vi "MOV_C-887.vi"(0 "System no.":i32=1 min=1 max=4 step=1, 2 "Axes to move":string[](array[string]), 3 "Position values":dbl[](array[numeric]) format="%.6f", 4 "No.of digits":i16=4, 5 "error in":errorcluster) -> (19 "error out":errorcluster)   [LabVIEW 2020]
doc: "GCS 3.0\n=====\n\nMOV (Start Absolute Motion)\n\nDescription\nSets absolute target positions for the specified axes and starts the motion to these target \npositions.\nAll axes specified in the command start the motion simultaneously.\nDuring motion, a new motion command sets the target to a new value and the old value may \nnever be reached.\n\nFormat\nMOV{ <AxisID> <Position>}\n\nArguments\n<AxisID>\nAn axis of the controller\nThe response to USG? CMD MOV indicates in the #Related Units block for which axes the \ncommand can be used.\nPossible values: Alias of the axis (p. 94) \n<Position>\nAbsolute target position in physical units\nThe data format is float.\nPossible values: Dependent on the permitted travel range of the axis\n\nResponse\nnone\n\nExample\n>>MOV?\n<<AXIS_1=0.0\n<<AXIS_2=0.0\n>>MOV AXIS_1 20 AXIS_2 40\n>>MOV?\n<<AXIS_1=20.000000000000000\n<<AXIS_2=40.000000000000000\n>>POS?\n<<AXIS_1=19.999494552\n<<AXIS_2=40.000494553\n\nNotes\nMotion is only executed if the following conditions are fulfilled for all specified axes:\n- The axis is in the Operation enabled state.\n- The mode of operation is set to Closed-Loop Position (0x2).\n- The target position is within the currently valid limits.\nFor further details, see \"Drive State Machine\" (p. 101) and the status register of the axis (p. 97). \nThe STV? command (p. 66) queries the status register.\nThe MOV command starts a motion and thus sets bit 18 \"In Motion\" of the status register of the \naxis. \nIf a new target position is set, the on-target state is reset to zero.\nThe MOV? command (p. 25) queries the currently valid target position.\nMotion can be stopped with the STP (p. 65) and HLT (p. 19) commands.\nThe travel range and the physical unit of the axis can be queried using the SPV? command\n(p. 63) with the following parameters:\n- AXIS_n - 0x121 ... Negative Soft Limit\n- AXIS_n - 0x122 ... Positive Soft Limit\n- AXIS_n - 0x106 ... Axis Metric Unit\nFor further information, see \"Motion Behavior - GCS 3.0\" (p. 101). \n\nUser command level\nUSR\n\n\nGCS 2.0\n=====\n\nMoves specified axes to specified absolute positions. No. of digits is the number of digits after the decimal point in the position value(s) that will be sent.\n\nC-413: Motion commands are not allowed when the wave generator is active or the analog input is used for target generation.\n\nC-867: This command works only in closed-loop operation. Motion commands like MOV are not allowed when a joystick is active on the axis.\n\nC-877: This command works only in closed-loop operation.\n\nC-880K005: VI only supported when called through PI_Multix.vi\n\nC-884: This command works only in closed-loop operation. Motion commands like MOV are not allowed when control via a Human Interface Device (HID) is active on the axis.\n\nC-885: This command works only in closed-loop operation.\n\nC-886: Motion commands are not allowed when a wave generator is active.\n\nC-891: This command works only in closed-loop operation. Motion commands are not allowed when the wave generator is active.\n\nE-517, E-518: Motion commands like MOV are not allowed when the controller is in OFFLINE mode or when the wave generator output is active. When a macro is running on the controller, MOV will be executed not until the macro is finished or stopped. See \"Control Value Generation\" and \"Control Modes\" in the controller user manual for details.\n\nE-709: Motion commands are not allowed when the wave generator is active or the analog input is used for target generation.\n\nE-712: Motion commands are not allowed when a wave generator is active or the analog input is used for target generation.\n\nE-725, E-727: Motion commands are not allowed when a wave generator is active or the analog input is used for target generation.\n\nE-753, E-754: Motion commands are not allowed when the wave generator is active or the analog input is used for target generation.\n\nE-755: Command not available for E-755.101.\n\nE-816: Only one axis per command allowed. It is necessary to wait a certain time before sending the next command to prevent it from being lost. \n\nE-861: This command works only in closed-loop operation. With open-loop systems, use OAD, OSM, OMA or OMR instead to command motion.\nMotion commands like MOV are not allowed when a joystick is active on the axis.\n\nE-871, E-873, E-874: This command works only in closed-loop operation. Motion commands like MOV are not allowed when a joystick is active on the axis.\n\nC-887, F-206, M-8X0: For GCS syntax version = GCS 1.0 (Check with CSV?.vi. If CSV?.vi is not supported, syntax version is GCS 1.0), no mix between F-206 axes X,Y,Z,U,V,W, separate axes A, B and NanoCube axes K, L, M in one call allowed. Subsequent MOV commands are handled in a buffer on controller, so please use General Wait for motion to stop.vi or #5.vi to check for motion to stop before sending the next MOV.\nFor GCS syntax version = GCS 2.0 or higher, subsequent MOV commands override the target position of the previous MOV command. Behavior can be changed by setting parameter 0x19001900 (SPA.vi), see controller user manual for details.\n\nHydra, Pollux: This command works only in closed-loop operation.\n\nMercury_GCS: This command works only in closed-loop operation. \nMotion commands like MOV are not allowed when a joystick is active on the axis."
panel:
  # "MOV (Start Absolute Motion)\n\nSets absolute target positions for the specified axes and starts the\nmotion to these target positions.\nAll axes specified in the command start the motion simultaneously.\nDuring motion, a new motion command sets the target to a new\nvalue and the old value may never be reached."
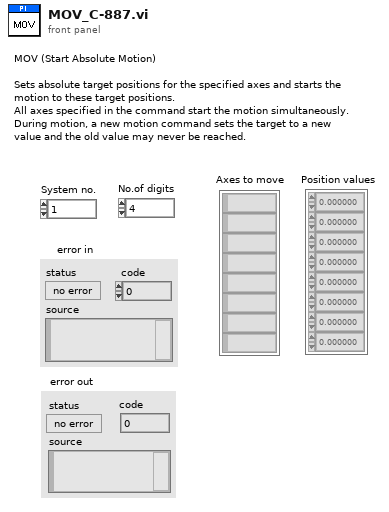
[diagram p1: front panel]
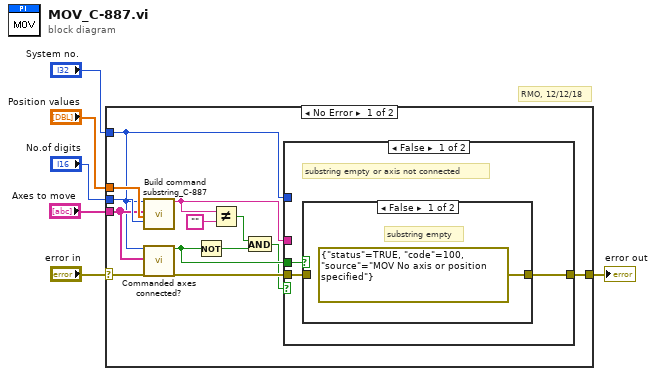
[diagram p0: block diagram]
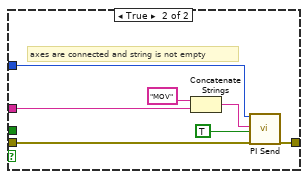
[diagram p3: hidden frame]
diagram:
  # "RMO, 12/12/18"
  n1 = case shown="No Error" "error in" {
    selector: "error in" -> [w7 w32]
    tunnel: [w19 w32] -> w6
    tunnel: "Position values" -> [w16 _]
    tunnel: "No.of digits" -> [w15 _]
    tunnel: "System no." -> [w8 _]
    tunnel: "Axes to move" -> [w13 _]
    frame No Error {
      n2 = call "Build command substring_C-887.vi"("System no."=w8, "Affected axes"=w13, "Parameters"=w16, "No. of digits"=w15) -> ("Command substring"=w17:string)  [unwired: 3 in, 12 out]
      n3 = call "Commanded axes connected?.vi"("System no."=w8, "Commanded axes"=w13, "error in"=w7) -> ("Controller error"=w11:bool, "error out"=w14:errorcluster)  [unwired: 1 in, 14 out]
      n4 = Not(x=w11) -> (.not. x?=w10:bool)
      n5 = Not Equal?(x=w17, y="") -> (x != y?=w12:bool)
      n6 = And(x=w12, y=w10) -> (x .and. y?=w9:bool)
      n7 = case shown="False" w9 {
        tunnel: w17 -> [_ w30]
        tunnel: [w22 w26] -> w19
        tunnel: w14 -> [w20 w27]
        tunnel: w11 -> [w21 _]
        tunnel: w8 -> [_ w25]
        frame False {
          # "substring empty or axis not connected"
          n8 = case shown="False" w21 {
            tunnel: [errorcluster {"status"=TRUE, "code"=100, "source"="MOV No axis or position specified"} ("error out") w24] -> w22
            tunnel: w20 -> [_ w24]
            frame False {
              # "substring empty"
            }
            frame True {
              # "commanded axis not connected"
            }
          }
        }
        frame True {
          # "axes are connected and string is not empty"
          n9 = Concatenate Strings("MOV", w30) -> (w28:string)
          n10 = call "PI Send.vi"("System no."=w25, "String to send"=w28, "Attach termination char.?"=TRUE ("Attach Linefeed?"), "error in"=w27) -> ("error out"=w26:errorcluster)  [unwired: 2 in, 13 out]
        }
      }
    }
    frame Error {
    }
  }
  "error out" <- w6
